vi "Save State As Default Helper.vi"(8 "Error In":errorcluster, 11 "Target VI":path) -> (0 "Error Out":errorcluster)   [LabVIEW 2014, in "LMH-Toolbox.lvlib" / "LMH-VITools.lvlib"]
uses:
  <vilib>/MakerHub/Toolbox/Private/VI Tools/LMH-VITools.lvlib
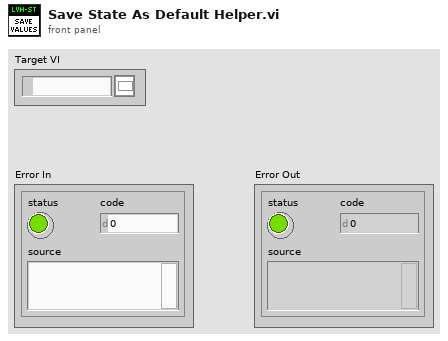
[diagram p1: front panel]
types:
  T1 = enum32{"Bad", "Idle", "Run top level", "Running"}
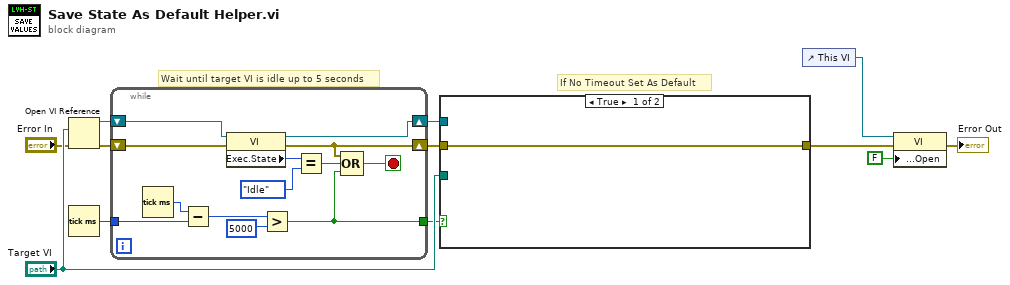
[diagram p0: block diagram]
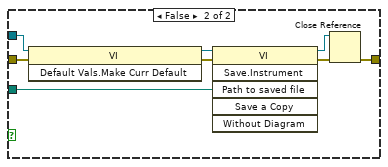
[diagram p2: hidden frame]
diagram:
  # "If No Timeout Set As Default"
  # "Wait until target VI is idle up to 5 seconds"
  n1 = Open VI Reference(vi path="Target VI", error in (no error)="Error In") -> (vi reference=w7:refnum<vi>, error out=w5:errorcluster)  [unwired: 4 in]
  n2 = Tick Count (ms)() -> (millisecond timer value=w4:u32)
  n3 = while {
    shift-right: [w24] -> w6
    shift-left: w7 -> [w25]
    shift-right: [w20] -> w2
    shift-left: w5 -> [w21]
    tunnel: w4 -> [w16]
    tunnel: [w13] -> w1
    stop <- w18 stop-if-true
    n4 = Tick Count (ms)() -> (millisecond timer value=w17:u32)
    n5 = Subtract(x=w17, y=w16) -> (x-y=w15:u32)
    n6 = property class="VI"(reference=w25, error in=w21) -> (reference out=w24:refnum<vi>, error out=w20:errorcluster, "Exec.State"=w23:T1)
    n7 = Greater?(x=w15, y=u32 5000) -> (0:w13:bool)
    n8 = Equal?(x=w23, y=T1."Idle") -> (x = y?=w19:bool)
    n9 = Compound Arithmetic op=OR(w20, w19, w13) -> (w18:bool)
  }
  n10 = case shown="True" w1 {
    tunnel: [w26 w32] -> w11
    tunnel: "Target VI" -> [_ w29]
    tunnel: w6 -> [_ w28]
    tunnel: w2 -> [w26 w27]
    frame True {
    }
    frame False {
      n11 = invoke class="VI" method="Default Vals.Make Curr Default"(reference=w28, error in=w27) -> (reference out=w31:refnum<vi>, error out=w30:errorcluster)  [unwired: 1 in, 1 out]
      n12 = invoke class="VI" method="Save.Instrument"(reference=w31, error in=w30, "Path to saved file"=w29) -> (reference out=w33:refnum<vi>, error out=w34:errorcluster)  [unwired: 3 in, 4 out]
      n13 = Close Reference(reference=w33, error in (no error)=w34) -> (error out=w32:errorcluster)
    }
  }
  n14 = control-ref of="This VI"() -> (w3:refnum<vi>)
  n15 = property class="VI"(reference=w3, error in=w11, "Front Panel Window:Open"=FALSE) -> (error out=→"Error Out":errorcluster)  [unwired: 1 out]
